vi "AutofocusInSession.vi"(2 "Method":T1=enum."Mean( Laplacian Convolution )", 3 "controller in":refnum<k24>, 4 "Session In":T2, 8 "Z position Guess":dbl=nan, 9 "error in (no error)":errorcluster) -> (0 "controller out":refnum<k24>, 1 "Session Out":T2, 5 "Autofocus Height":dbl, 6 "error out":errorcluster, 7 "Total Images":i32)   [LabVIEW 2016]
doc: "Peroforms an AutoFocus height setting procedure on the spot, using the fitting techniques used in the 1_2_UnifiedCameraCalibration VI. By fitting after each image, however, this VI can dynamically adjust its list of locations to test contrast at based on the fit on the previous locations, using the following pattern:\nFirst, 5 images are taken, spaced by 1mm each, ranging from 2mm above to 2mm below the initial guess. The 5 points are then fitted, and each subsequent guess is either at the predicted focus height, or exteending the range by another 1mm if the predicted focus height is outside the range of the previous data points."
uses:
  C:/Users/sciollalab/Documents/Brandeis-BNL/LabVIEW_Codes/BNLStaveAssembly-Blueprint/Bin/Aerotech.A3200.dll
  BNLStaveAssembly-Blueprint/Bin/Aerotech.A3200.dll
  <vilib>/userdefined/High Color/IMAQdx.ctl
  Controls/All_Enums/Enum_TypeDef_ImageSharpnessAnalysisMethod.ctl
  <vilib>/vision/driver/NI_Vision_Acquisition_Software.lvlib
panel:
  in  "Tolerance":dbl=0.03 format="%#_13g"
  in  "Step Size":dbl=1.0 format="%#_13g"
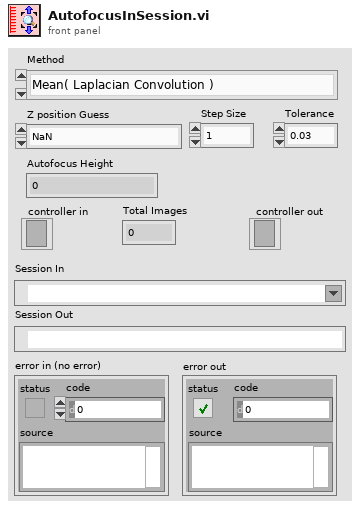
[diagram p1: front panel]
types:
  T1 = typedef "Enum_TypeDef_ImageSharpnessAnalysisMethod.ctl" = enum16{"sigma( Intensity )", "Mean( Laplacian Convolution )"}
  T2 = typedef "IMAQdx.ctl" = refnum<k21>
  T3 = cluster{"vX [mm/s]":dbl, "vY [mm/s]":dbl, "vZ [mm/s]":dbl}
  T4 = cluster{"X Position Feedback":dbl, "Y Position Feedback":dbl, "Z Position Feedback":dbl}
  T5 = typedef "IMAQ Image.ctl" = refnum<image>
  T6 = cluster{"Final X":dbl, "Final Y":dbl, "Final Z":dbl}
  T7 = cluster{dbl[], dbl[], dbl[], "Max Out":dbl, "Min Out":dbl}
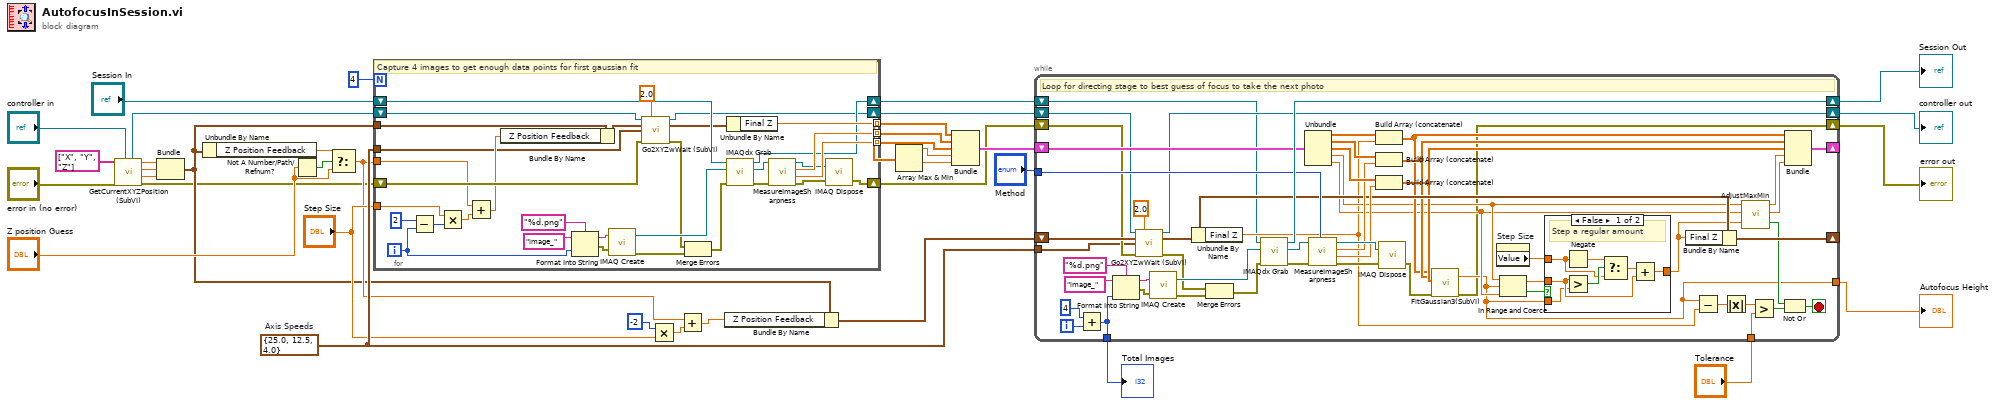
[diagram p0: block diagram]
diagram:
  w20 = T3 {"vX [mm/s]"=25.0, "vY [mm/s]"=12.5, "vZ [mm/s]"=4.0}  # Axis Speeds
  n1 = call "GetCurrentXYZPosition (SubVI).vi"(".NET Refnum in - Device"="controller in", "error in (no error)"="error in (no error)", "Axes Names"=string[] ["X", "Y", "Z"]) -> ("error out"=w6:errorcluster, "Z Position Feedback"=w24:dbl, "Y Position Feedback"=w25:dbl, "X Position Feedback"=w26:dbl, ".NET Refnum out  - Device"=w1:refnum<k24>)  [unwired: 3 in, 1 out]
  n2 = Bundle("X Position Feedback"=w26, "Y Position Feedback"=w25, "Z Position Feedback"=w24) -> (w10:T4)  [unwired: 1 in]
  n3 = Unbundle By Name(w10) -> ("Z Position Feedback"=w22:dbl)
  n4 = Not A Number/Path/Refnum?(number/path/refnum="Z position Guess") -> (NaN/Path/Refnum?=w23:bool)
  n5 = Select(t=w22, s=w23, f="Z position Guess") -> (s? t:f=w11:dbl)
  n6 = for {
    N: 4 -> [_]
    tunnel: w11 -> [w48]
    tunnel: w10 -> [w58]
    tunnel: [w56] -> w18 mode=indexing
    tunnel: [w55] -> w17 mode=indexing
    shift-right: [w43] -> w3
    shift-left: w6 -> [w54]
    tunnel: "Step Size" -> [w50]
    tunnel: [w45] -> w19 mode=indexing
    shift-right: [w41] -> w5
    shift-left: "Session In" -> [w59]
    tunnel: w20 -> [w40]
    shift-right: [w39] -> w4
    shift-left: w1 -> [w38]
    i -> [w53]
    # "Capture 4 images to get enough data points for first gaussian fit"
    n7 = Subtract(x=2, y=w53) -> (x-y=w51:i32)
    n8 = Multiply(x=w50, y=w51) -> (x*y=w49:dbl)
    n9 = Add(x=w48, y=w49) -> (x+y=w47:dbl)
    n10 = Bundle By Name(cluster=w58, "Z Position Feedback"=w47) -> (w57:T4)
    n11 = Format Into String(format string="%d.png", initial string="image_", w53) -> (resulting string=w68:string, error out=w67:errorcluster)  [unwired: 1 in]
    n12 = call "IMAQ Create"("Image Name"=w68, "error in (no error)"=w67) -> ("New Image"=w66:T5, "error out"=w62:errorcluster)  [unwired: 2 in, 1 out]
    n13 = call "Go2XYZwWait (SubVI).vi"(".NET Refnum in"=w38, "Delay Time (s)"=2.0, "Go to Coordinates"=w57, "Axis Speeds"=w40, "error in (no error)"=w54) -> (".NET Refnum out"=w39:refnum<k24>, "Final Position"=w46:T6, "error out"=w63:errorcluster)  [unwired: 6 in, 2 out]
    n14 = Merge Errors(w63, w62) -> (w61:errorcluster)
    n15 = Unbundle By Name(w46) -> ("Final Z"=w45:dbl)
    n16 = call <vilib>:"IMAQdx Grab.vi"("error in"=w61, "Image In"=w66, "Session In"=w59) -> ("error out"=w64:errorcluster, "Image Out"=w65:T5, "Session Out"=w41:T2)  [unwired: 1 in, 5 out]
    n17 = call "MeasureImageSharpness.vi"("error in (no error)"=w64, "Image In"=w65) -> ("error out"=w44:errorcluster, "Sharpness Uncertainty"=w55:dbl, "Sharpness"=w56:dbl, "Image Out"=w42:T5)  [unwired: 6 in]
    n18 = call "IMAQ Dispose"("Image"=w42, "error in (no error)"=w44) -> ("error out"=w43:errorcluster)  [unwired: 4 in]
  }
  n19 = Multiply(x=-2, y="Step Size") -> (x*y=w12:dbl)
  n20 = Add(x=w11, y=w12) -> (x+y=w9:dbl)
  n21 = Bundle By Name(cluster=w10, "Z Position Feedback"=w9) -> (w8:T4)
  n22 = Array Max & Min(array=w19) -> (max value=w16:dbl, min value=w15:dbl)  [unwired: 2 out]
  n23 = Bundle(w19, w18, w17, w16, w15) -> (w7:cluster{dbl[], dbl[], dbl[], dbl, dbl})  [unwired: 1 in]
  n24 = while {
    tunnel: "Method" -> [w114]
    shift-right: [w92] -> _
    shift-left: w7 -> [w108]
    shift-right: [w101] -> _
    shift-left: w8 -> [w100]
    tunnel: "Tolerance" -> [w86]
    tunnel: [w73] -> w34
    shift-right: [w71] -> w32
    shift-left: w3 -> [w81]
    shift-right: [w80] -> w31
    shift-left: w4 -> [w79]
    tunnel: [w78] -> w30
    tunnel: w20 -> [w76]
    shift-right: [w117] -> w33
    shift-left: w5 -> [w75]
    i -> [w122]
    stop <- w83 stop-if-true
    # "Loop for directing stage to best guess of focus to take the next photo"
    n25 = Add(x=4, y=w122) -> (x+y=w78:i32)
    n26 = Format Into String(format string="%d.png", initial string="image_", w78) -> (resulting string=w120:string, error out=w119:errorcluster)  [unwired: 1 in]
    n27 = call "Go2XYZwWait (SubVI).vi"(".NET Refnum in"=w79, "Delay Time (s)"=2.0, "Go to Coordinates"=w100, "Axis Speeds"=w76, "error in (no error)"=w81) -> (".NET Refnum out"=w80:refnum<k24>, "Final Position"=w102:T6, "error out"=w111:errorcluster)  [unwired: 6 in, 2 out]
    n28 = call "IMAQ Create"("Image Name"=w120, "error in (no error)"=w119) -> ("New Image"=w118:T5, "error out"=w110:errorcluster)  [unwired: 2 in, 1 out]
    n29 = Unbundle By Name(w102) -> ("Final Z"=w85:dbl)
    n30 = Merge Errors(w111, w110) -> (w109:errorcluster)
    n31 = call <vilib>:"IMAQdx Grab.vi"("error in"=w109, "Image In"=w118, "Session In"=w75) -> ("error out"=w115:errorcluster, "Image Out"=w116:T5, "Session Out"=w117:T2)  [unwired: 1 in, 5 out]
    n32 = Unbundle(w108) -> (w107:dbl[], w105:dbl[], w106:dbl[], w94:dbl, w93:dbl)
    n33 = call "MeasureImageSharpness.vi"("Method"=w114, "error in (no error)"=w115, "Image In"=w116) -> ("error out"=w112:errorcluster, "Sharpness Uncertainty"=w103:dbl, "Sharpness"=w104:dbl, "Image Out"=w113:T5)  [unwired: 5 in]
    n34 = Build Array (concatenate)(w107, w85) -> (w97:dbl[])
    n35 = Build Array (concatenate)(w105, w104) -> (w98:dbl[])
    n36 = Build Array (concatenate)(w106, w103) -> (w99:dbl[])
    n37 = call "IMAQ Dispose"("Image"=w113, "error in (no error)"=w112) -> ("error out"=w72:errorcluster)  [unwired: 4 in]
    n38 = call "FitGaussian3(SubVI).vi"("x values"=w97, "y values"=w98, "delta y values"=w99, "error in"=w72) -> ("Optimized position"=w73:dbl, "error out"=w71:errorcluster)  [unwired: 10 in, 4 out]
    n39 = property on="Step Size" class="DigNum (strict)"() -> ("Value"=w74:dbl)  [unwired: 2 in, 2 out]
    n40 = In Range and Coerce(upper limit=w94, x=w73, lower limit=w93) -> (coerced(x)=w96:dbl, In Range?=w95:bool)
    n41 = case shown="False" w95 {
      tunnel: [w128 w132] -> w89
      tunnel: w96 -> [w126 w132]
      tunnel: w74 -> [w129 _]
      tunnel: w73 -> [w125 _]
      frame False {
        # "Step a regular amount"
        n42 = Negate(x=w129) -> (-x=w131:dbl)
        n43 = Greater?(x=w126, y=w125) -> (0:w130:bool)
        n44 = Select(t=w131, s=w130, f=w129) -> (s? t:f=w127:dbl)
        n45 = Add(x=w127, y=w126) -> (x+y=w128:dbl)
      }
      frame True {
        # "Go to best guess"
      }
    }
    n46 = Bundle By Name(cluster=w102, "Final Z"=w89) -> (w101:T6)
    n47 = Subtract(x=w73, y=w85) -> (x-y=w88:dbl)
    n48 = Absolute Value(x=w88) -> (abs(x)=w87:dbl)
    n49 = call "AdjustMaxMin.vi"("Max In"=w94, "Min In"=w93, "Input"=w89) -> ("Max Out"=w90:dbl, "Min Out"=w91:dbl, "Bounds Extended"=w82:bool)  [unwired: 1 in]
    n50 = Greater?(x=w87, y=w86) -> (0:w84:bool)
    n51 = Not Or(1:w84, 2:w82) -> (0:w83:bool)
    n52 = Bundle(w97, w98, w99, "Max Out"=w90, "Min Out"=w91) -> (w92:T7)  [unwired: 1 in]
  }
  "controller out" <- w31
  "Session Out" <- w33
  "Autofocus Height" <- w34
  "error out" <- w32
  "Total Images" <- w30
